vi "Read Read Only.vi"(8 "error in (no error)":errorcluster, 11 "Const_I32 in":refnum<class "Const_I32.lvclass">) -> (0 "error out":errorcluster, 2 "Read Only":bool, 3 "Const_I32 out":refnum<class "Const_I32.lvclass">)   [LabVIEW 2021, in "Const_I32.lvclass"]
uses:
  Const_I32.lvclass
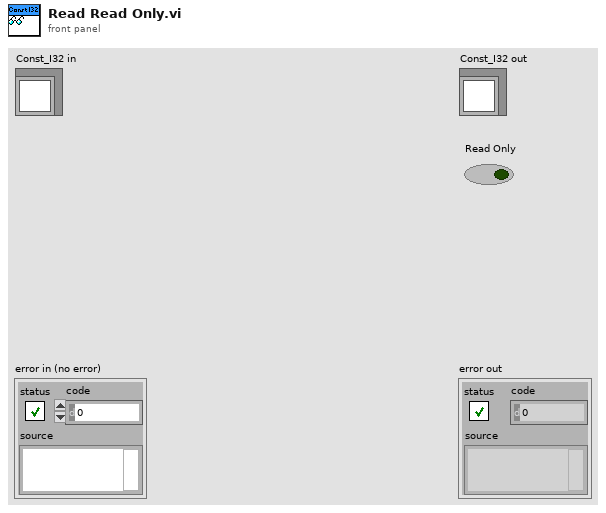
[diagram p1: front panel]
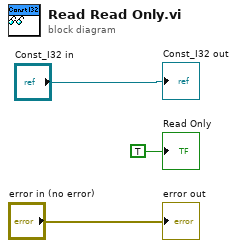
[diagram p0: block diagram]
diagram:
  "error out" <- "error in (no error)"
  "Const_I32 out" <- "Const_I32 in"
  "Read Only" <- TRUE ("Read Only")
